vi "Divide SGL - Kintex7.vi"(0 "A":sgl, 1 "B":sgl, 3 "Data Valid In":bool=TRUE) -> (7 "Result":sgl, 10 "Data Valid Out":bool)   [LabVIEW 2014]
uses:
  <vilib>/rvi/XilinxIP/XIPIN_XNode/niFpgaXIPIN.xnode
  DivideSGL_K7/xsim.dir/DivideSGL_K7_EB72A9E93DBE4CEBB2626B44969B07DB/xsimk_EB72A9E93DBE4CEBB2626B44969B07DB.dll
  <vilib>/rvi/IPIntegrationNode/IPINode_Xnode/niFpgaIPINode.xnode
  <vilib>/rvi/IPIntegrationNode/IPINode_Typedef/niFpgaIPINodeSupportedFamilies.ctl
  <vilib>/rvi/IPIntegrationNode/IPINode_Utilities/niFpgaIPINodeSimCore.vi
panel:
  # "Copyright 2014 Vidrio Technologies\nScanImage 5 software is licensed under the Apache License, Version 2.0 (the \"License\"); you may not use any files contained\nwithin the ScanImage 5 release except in compliance with the License. You may obtain a copy of the License at\n http://www.apache.org/licenses/LICENSE-2.0\nUnless required by applicable law or agreed to in writing, software distributed under the License is distributed on an\n\"AS IS\" BASIS, WITHOUT WARRANTIES OR CONDITIONS OF ANY KIND, either express or implied. See the License for the\n specific language governing permissions and limitations under the License."
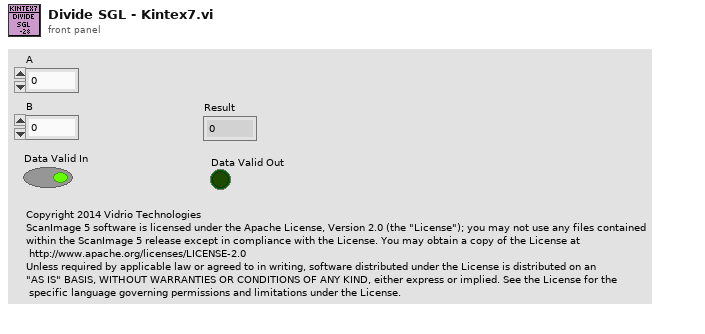
[diagram p1: front panel]
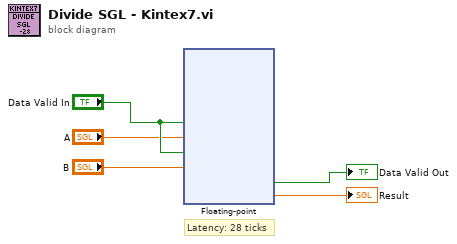
[diagram p0: block diagram]
diagram:
  # "Latency: 28 ticks"
  n1 = xnode ("Floating-point")("s_axis_a_tvalid"="Data Valid In", "s_axis_a_tdata"="A", "s_axis_b_tvalid"="Data Valid In", "s_axis_b_tdata"="B") -> ("m_axis_result_tvalid"=→"Data Valid Out":bool, "m_axis_result_tdata"=→"Result":sgl)
